vi "write_txt_string.vi"(8 "error in (no error)":errorcluster, 10 "data string":string, 11 "DataLoggingText in":refnum<class "DataLogging.lvclass">) -> (0 "error out":errorcluster, 3 "DataLoggingText out":refnum<class "DataLogging.lvclass">)   [LabVIEW 2018, in "DataLogging.lvclass"]
doc: "writes data into a text file.\ndata are:\n- any string"
uses:
  DataLogging.lvclass
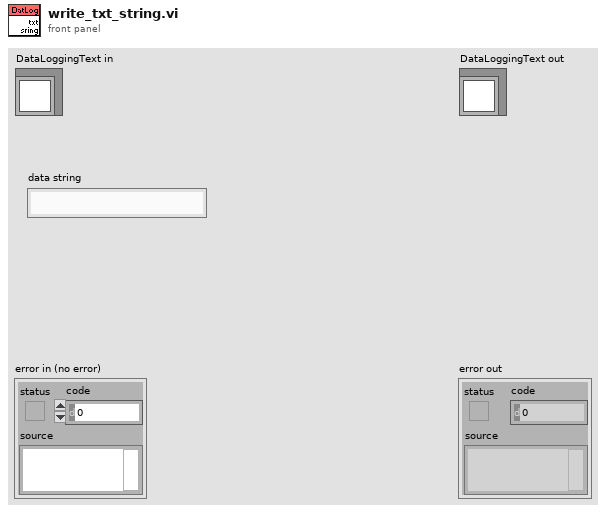
[diagram p1: front panel]
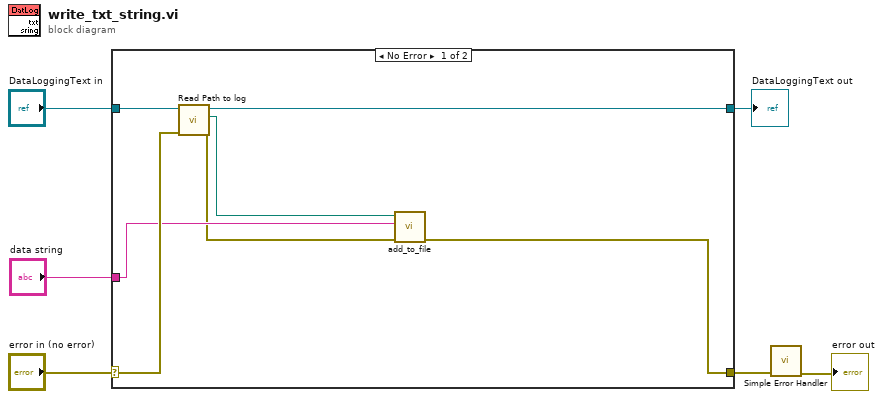
[diagram p0: block diagram]
diagram:
  n1 = case shown="No Error" "error in (no error)" {
    selector: "error in (no error)" -> [w12 w15]
    tunnel: [w7 w15] -> w2
    tunnel: [w11 w14] -> w4
    tunnel: "DataLoggingText in" -> [w13 w14]
    tunnel: "data string" -> [w9 _]
    frame No Error {
      n2 = call-dynamic "Read Path to log.vi"("error in (no error)"=w12, "DataLoggingText in"=w13) -> ("error out"=w8:errorcluster, "Path to log"=w10:path, "DataLoggingText out"=w11:refnum<class "DataLogging.lvclass">)  [unwired: 7 in]
      n3 = call "add_to_file.vi"("error in (no error)"=w8, "String"=w9, "Path to log"=w10) -> ("error out"=w7:errorcluster)  [unwired: 8 in]
    }
    frame Error {
    }
  }
  "DataLoggingText out" <- w4
  n4 = call <vilib>:"Simple Error Handler.vi"("error in (no error)"=w2) -> ("error out"=→"error out":errorcluster)  [unwired: 4 in, 4 out]
